vi "test_read-nmea-data2.vi"() -> ()   [LabVIEW 2019] (continued)
F9P\t\t\n15:10:07.17\tF9P\t\t\n15:10:07.19\tF9P\t\t\n15:10:07.21\tF9P\t\t\n15:10:07.23\tF9P\t\t\n15:10:07.25\tF9P\t$GNRMC,061009.00,A,3723.58159,N,12656.88383,E,1.806,,250720,,,A,V*1C\n\t\n15:10:07.27\tF9P\t$GNVTG,,T,,M,1.806,N,3.344,K,A*32\n\t\n15:10:07.29\tF9P\t$GNGGA,061009.00,3723.58159,N,12656.88383,E,1,12,0.64,44.5,M,18.5,M,,*7F\n\t\n15:10:07.31\tF9P\t$GNGSA,A,3,12,06,19,05,17,09,04,02,,,,,1.19,0.64,1.00,1*0A\n\t\n15:10:07.33\tF9P\t$GNGSA,A,3,85,71,84,,,,,,,,,,1.19,0.64,1.00,2*0F\n\t\n15:10:07.35\tF9P\t$GNGSA,A,3,36,19,11,04,09,12,,,,,,,1.19,0.64,1.00,3*0A\n\t\n15:10:07.37\tF9P\t$GNGSA,A,3,14,11,33,,,,,,,,,,1.19,0.64,1.00,4*0B\n\t\n15:10:07.39\tF9P\t$GPGSV,3,1,09,02,54,318,25,04,19,044,11,05,36,246,25,06,65,046,30,1*6E\n\t\n15:10:07.41\tF9P\t$GPGSV,3,2,09,09,45,075,26,12,24,278,18,17,34,153,25,19,53,156,23,1*6F\n\t\n15:10:07.43\tF9P\t$GPGSV,3,3,09,25,12,307,15,1*59\n\t\n15:10:07.45\tF9P\t$GPGSV,3,1,09,02,54,318,,04,19,044,,05,36,246,18,06,65,046,13,6*61\n\t\n15:10:07.47\tF9P\t$GPGSV,3,2,09,09,45,075,12,12,24,278,,17,34,153,,19,53,156,,6*60\n\t\n15:10:07.49\tF9P\t$GPGSV,3,3,09,25,12,307,,6*5A\n\t\n15:10:07.51\tF9P\t$GLGSV,2,1,08,69,12,031,,70,72,041,,71,51,205,19,72,03,209,,1*7A\n\t\n15:10:07.53\tF9P\t$GLGSV,2,2,08,77,01,327,,84,21,121,11,85,70,063,21,86,35,329,,1*76\n\t\n15:10:07.55\tF9P\t$GLGSV,2,1,08,69,12,031,,70,72,041,,71,51,205,28,72,03,209,,3*7A\n\t\n15:10:07.57\tF9P\t$GLGSV,2,2,08,77,01,327,,84,21,121,14,85,70,063,20,86,35,329,,3*70\n\t\n15:10:07.59\tF9P\t$GAGSV,2,1,08,02,09,298,10,04,66,119,24,09,31,193,15,11,71,357,22,7*79\n\t\n15:10:07.61\tF9P\t$GAGSV,2,2,08,12,40,102,18,19,27,045,22,25,09,249,,36,25,308,16,7*75\n\t\n15:10:07.63\tF9P\t$GAGSV,2,1,08,02,09,298,,04,66,119,20,09,31,193,,11,71,357,15,2*79\n\t\n15:10:07.65\tF9P\t$GAGSV,2,2,08,12,40,102,,19,27,045,,25,09,249,,36,25,308,,2*7E\n\t\n15:10:07.67\tF9P\t$GBGSV,1,1,03,11,50,131,19,14,87,138,20,33,60,219,25,1*42\n\t\n15:10:07.69\tF9P\t$GBGSV,1,1,03,11,50,131,16,14,87,138,22,33,60,219,,3*4A\n\t\n15:10:07.71\tF9P\t$GNGLL,3723.58159,N,12656.88383,E,061009.00,A,A*72\n\t\n15:10:07.73\tF9P\t\t\n15:10:07.75\tF9P\t\t\n15:10:07.77\tF9P\t\t\n15:10:07.79\tF9P\t\t\n15:10:07.81\tF9P\t\t\n15:10:07.83\tF9P\t\t\n15:10:07.85\tF9P\t\t\n15:10:07.87\tF9P\t\t\n15:10:07.89\tF9P\t\t\n15:10:07.91\tF9P\t\t\n15:10:07.93\tF9P\t\t\n15:10:07.95\tF9P\t\t\n15:10:07.97\tF9P\t\t\n15:10:07.99\tF9P\t\t\n15:10:08.01\tF9P\t\t\n15:10:08.03\tF9P\t\t\n15:10:08.05\tF9P\t\t\n15:10:08.07\tF9P\t\t\n15:10:08.09\tF9P\t\t\n15:10:08.11\tF9P\t\t\n15:10:08.13\tF9P\t\t\n15:10:08.15\tF9P\t\t\n15:10:08.17\tF9P\t\t\n15:10:08.19\tF9P\t\t\n15:10:08.21\tF9P\t\t\n15:10:08.23\tF9P\t\t\n15:10:08.25\tF9P\t$GNRMC,061010.00,A,3723.58119,N,12656.88346,E,1.587,,250720,,,A,V*1D\n\t\n15:10:08.27\tF9P\t$GNVTG,,T,,M,1.587,N,2.938,K,A*36\n\t\n15:10:08.29\tF9P\t$GNGGA,061010.00,3723.58119,N,12656.88346,E,1,12,0.64,46.1,M,18.5,M,,*7C\n\t\n15:10:08.31\tF9P\t$GNGSA,A,3,12,06,19,05,17,09,04,02,,,,,1.19,0.64,1.00,1*0A\n\t\n15:10:08.33\tF9P\t$GNGSA,A,3,85,71,84,,,,,,,,,,1.19,0.64,1.00,2*0F\n\t\n15:10:08.35\tF9P\t$GNGSA,A,3,36,19,11,04,09,12,,,,,,,1.19,0.64,1.00,3*0A\n\t\n15:10:08.37\tF9P\t$GNGSA,A,3,14,11,33,,,,,,,,,,1.19,0.64,1.00,4*0B\n\t\n15:10:08.39\tF9P\t$GPGSV,3,1,09,02,54,318,24,04,19,044,14,05,36,246,24,06,65,046,25,1*6F\n\t\n15:10:08.41\tF9P\t$GPGSV,3,2,09,09,45,075,33,12,24,278,19,17,34,153,23,19,53,156,23,1*6C\n\t\n15:10:08.43\tF9P\t$GPGSV,3,3,09,25,12,307,14,1*58\n\t\n15:10:08.45\tF9P\t$GPGSV,3,1,09,02,54,318,,04,19,044,,05,36,246,17,06,65,046,15,6*68\n\t\n15:10:08.47\tF9P\t$GPGSV,3,2,09,09,45,075,12,12,24,278,,17,34,153,,19,53,156,,6*60\n\t\n15:10:08.49\tF9P\t$GPGSV,3,3,09,25,12,307,,6*5A\n\t\n15:10:08.51\tF9P\t$GLGSV,2,1,08,69,12,031,,70,72,041,,71,51,205,18,72,03,209,,1*7B\n\t\n15:10:08.53\tF9P\t$GLGSV,2,2,08,77,01,327,,84,21,121,10,85,70,063,21,86,35,329,,1*77\n\t\n15:10:08.55\tF9P\t$GLGSV,2,1,08,69,12,031,,70,72,041,,71,51,205,27,72,03,209,,3*75\n\t\n15:10:08.57\tF9P\t$GLGSV,2,2,08,77,01,327,,84,21,121,13,85,70,063,20,86,35,329,,3*77\n\t\n15:10:08.59\tF9P\t$GAGSV,2,1,08,02,09,298,10,04,66,119,26,09,31,193,19,11,71,357,21,7*74\n\t\n15:10:08.61\tF9P\t$GAGSV,2,2,08,12,40,102,20,19,27,045,24,25,09,249,,36,25,308,18,7*76\n\t\n15:10:08.63\tF9P\t$GAGSV,2,1,08,02,09,298,,04,66,119,20,09,31,193,,11,71,357,16,2*7A\n\t\n15:10:08.65\tF9P\t$GAGSV,2,2,08,12,40,102,,19,27,045,,25,09,249,,36,25,308,,2*7E\n\t\n15:10:08.67\tF9P\t$GBGSV,1,1,03,11,50,131,19,14,87,138,21,33,60,219,26,1*40\n\t\n15:10:08.69\tF9P\t$GBGSV,1,1,03,11,50,131,18,14,87,138,22,33,60,219,,3*44\n\t\n15:10:08.71\tF9P\t$GNGLL,3723.58119,N,12656.88346,E,061010.00,A,A*77\n\t\n15:10:08.74\tF9P\t\t\n15:10:08.76\tF9P\t\t\n15:10:08.78\tF9P\t\t\n15:10:08.80\tF9P\t\t\n15:10:08.82\tF9P\t\t\n15:10:08.84\tF9P\t\t\n15:10:08.86\tF9P\t\t\n15:10:08.88\tF9P\t\t\n15:10:08.90\tF9P\t\t\n15:10:08.92\tF9P\t\t\n15:10:08.94\tF9P\t\t\n15:10:08.96\tF9P\t\t\n15:10:08.98\tF9P\t\t\n15:10:09.00\tF9P\t\t\n15:10:09.02\tF9P\t\t\n15:10:09.04\tF9P\t\t\n15:10:09.06\tF9P\t\t\n15:10:09.08\tF9P\t\t\n15:10:09.10\tF9P\t\t\n15:10:09.12\tF9P\t\t\n15:10:09.14\tF9P\t\t\n15:10:09.16\tF9P\t\t\n15:10:09.18\tF9P\t\t\n15:10:09.20\tF9P\t\t\n15:10:09.22\tF9P\t\t\n15:10:09.24\tF9P\t\t\n15:10:09.26\tF9P\t$GNRMC,061011.00,A,3723.58042,N,12656.88317,E,2.775,203.67,250720,,,A,V*05\n\t\n15:10:09.28\tF9P\t$GNVTG,203.67,T,,M,2.775,N,5.139,K,A*2A\n\t\n15:10:09.30\tF9P\t$GNGGA,061011.00,3723.58042,N,12656.88317,E,1,12,0.64,47.7,M,18.5,M,,*71\n\t\n15:10:09.32\tF9P\t$GNGSA,A,3,12,06,19,05,17,09,04,02,,,,,1.19,0.64,1.00,1*0A\n\t\n15:10:09.34\tF9P\t$GNGSA,A,3,85,71,84,,,,,,,,,,1.19,0.64,1.00,2*0F\n\t\n15:10:09.36\tF9P\t$GNGSA,A,3,36,19,11,04,09,12,,,,,,,1.19,0.64,1.00,3*0A\n\t\n15:10:09.38\tF9P\t$GNGSA,A,3,14,11,33,,,,,,,,,,1.19,0.64,1.00,4*0B\n\t\n15:10:09.40\tF9P\t$GPGSV,3,1,09,02,54,318,23,04,19,044,14,05,36,246,24,06,65,046,32,1*6E\n\t\n15:10:09.42\tF9P\t$GPGSV,3,2,09,09,45,075,33,12,24,278,18,17,34,153,23,19,53,156,24,1*6A\n\t\n15:10:09.44\tF9P\t$GPGSV,3,3,09,25,12,307,13,1*5F\n\t\n15:10:09.46\tF9P\t$GPGSV,3,1,09,02,54,318,,04,19,044,,05,36,246,18,06,65,046,15,6*67\n\t\n15:10:09.48\tF9P\t$GPGSV,3,2,09,09,45,075,,12,24,278,,17,34,153,,19,53,156,,6*63\n\t\n15:10:09.50\tF9P\t$GPGSV,3,3,09,25,12,307,,6*5A\n\t\n15:10:09.52\tF9P\t$GLGSV,2,1,08,69,12,031,,70,72,041,,71,51,205,18,72,03,209,,1*7B\n\t\n15:10:09.54\tF9P\t$GLGSV,2,2,08,77,01,327,,84,21,121,10,85,70,063,22,86,35,329,,1*74\n\t\n15:10:09.56\tF9P\t$GLGSV,2,1,08,69,12,031,,70,72,041,,71,51,205,26,72,03,209,,3*74\n\t\n15:10:09.58\tF9P\t$GLGSV,2,2,08,77,01,327,,84,21,121,18,85,70,063,20,86,35,329,,3*7C\n\t\n15:10:09.60\tF9P\t$GAGSV,2,1,08,02,09,298,10,04,66,119,26,09,31,193,19,11,71,357,21,7*74\n\t\n15:10:09.62\tF9P\t$GAGSV,2,2,08,12,40,102,21,19,27,045,24,25,09,249,,36,25,308,17,7*78\n\t\n15:10:09.64\tF9P\t$GAGSV,2,1,08,02,09,298,,04,66,119,20,09,31,193,,11,71,357,14,2*78\n\t\n15:10:09.66\tF9P\t$GAGSV,2,2,08,12,40,102,,19,27,045,,25,09,249,,36,25,308,,2*7E\n\t\n15:10:09.68\tF9P\t$GBGSV,1,1,03,11,50,131,18,14,87,138,20,33,60,219,26,1*40\n\t\n15:10:09.70\tF9P\t$GBGSV,1,1,03,11,50,131,18,14,87,138,21,33,60,219,,3*47\n\t\n15:10:09.72\tF9P\t$GNGLL,3723.58042,N,12656.88317,E,061011.00,A,A*7D\n\t\n15:10:09.74\tF9P\t\t\n15:10:09.76\tF9P\t\t\n15:10:09.78\tF9P\t\t\n15:10:09.80\tF9P\t\t\n15:10:09.82\tF9P\t\t\n15:10:09.84\tF9P\t\t\n15:10:09.86\tF9P\t\t\n15:10:09.88\tF9P\t\t\n15:10:09.90\tF9P\t\t\n15:10:09.92\tF9P\t\t\n15:10:09.94\tF9P\t\t\n15:10:09.96\tF9P\t\t\n15:10:09.98\tF9P\t\t\n15:10:10.00\tF9P\t\t\n15:10:10.02\tF9P\t\t\n15:10:10.04\tF9P\t\t\n15:10:10.06\tF9P\t\t\n15:10:10.08\tF9P\t\t\n15:10:10.10\tF9P\t\t\n15:10:10.12\tF9P\t\t\n15:10:10.14\tF9P\t\t\n15:10:10.16\tF9P\t\t\n15:10:10.18\tF9P\t\t\n15:10:10.20\tF9P\t\t\n15:10:10.22\tF9P\t\t\n15:10:10.24\tF9P\t\t\n15:10:10.26\tF9P\t$GNRMC,061012.00,A,3723.57986,N,12656.88305,E,1.614,,250720,,,A,V*10\n\t\n15:10:10.28\tF9P\t$GNVTG,,T,,M,1.614,N,2.989,K,A*35\n\t\n15:10:10.30\tF9P\t$GNGGA,061012.00,3723.57986,N,12656.88305,E,1,12,0.64,49.2,M,18.5,M,,*74\n\t\n15:10:10.32\tF9P\t$GNGSA,A,3,12,06,19,05,17,09,04,02,,,,,1.19,0.64,1.00,1*0A\n\t\n15:10:10.34\tF9P\t$GNGSA,A,3,85,71,84,,,,,,,,,,1.19,0.64,1.00,2*0F\n\t\n15:10:10.36\tF9P\t$GNGSA,A,3,36,19,11,04,09,12,,,,,,,1.19,0.64,1.00,3*0A\n\t\n15:10:10.38\tF9P\t$GNGSA,A,3,14,11,33,,,,,,,,,,1.19,0.64,1.00,4*0B\n\t\n15:10:10.40\tF9P\t$GPGSV,3,1,09,02,54,318,22,04,19,044,14,05,36,246,24,06,65,046,31,1*6C\n\t\n15:10:10.42\tF9P\t$GPGSV,3,2,09,09,45,075,20,12,24,278,19,17,34,153,22,19,53,156,22,1*6E\n\t\n15:10:10.44\tF9P\t$GPGSV,3,3,09,25,12,307,12,1*5E\n\t\n15:10:10.46\tF9P\t$GPGSV,3,1,09,02,54,318,,04,19,044,,05,36,246,18,06,65,046,16,6*64\n\t\n15:10:10.48\tF9P\t$GPGSV,3,2,09,09,45,075,,12,24,278,,17,34,153,,19,53,156,,6*63\n\t\n15:10:10.50\tF9P\t$GPGSV,3,3,09,25,12,307,,6*5A\n\t\n15:10:10.52\tF9P\t$GLGSV,2,1,08,69,12,031,,70,72,041,,71,51,205,17,72,03,209,,1*74\n\t\n15:10:10.54\tF9P\t$GLGSV,2,2,08,77,01,327,,84,21,121,10,85,70,063,23,86,35,329,,1*75\n\t\n15:10:10.56\tF9P\t$GLGSV,2,1,08,69,12,031,,70,72,041,,71,51,205,24,72,03,209,,3*76\n\t\n15:10:10.58\tF9P\t$GLGSV,2,2,08,77,01,327,,84,21,121,14,85,70,063,19,86,35,329,,3*7A\n\t\n15:10:10.60\tF9P\t$GAGSV,2,1,08,02,09,298,08,04,66,119,31,09,31,193,19,11,71,357,22,7*78\n\t\n15:10:10.62\tF9P\t$GAGSV,2,2,08,12,40,102,20,19,27,045,23,25,09,249,,36,25,308,18,7*71\n\t\n15:10:10.64\tF9P\t$GAGSV,2,1,08,02,09,298,,04,66,119,21,09,31,193,,11,71,357,15,2*78\n\t\n15:10:10.66\tF9P\t$GAGSV,2,2,08,12,40,102,,19,27,045,,25,09,249,,36,25,308,,2*7E\n\t\n15:10:10.68\tF9P\t$GBGSV,1,1,03,11,50,131,20,14,87,138,19,33,60,219,26,1*41\n\t\n15:10:10.70\tF9P\t$GBGSV,1,1,03,11,50,131,28,14,87,138,20,33,60,219,,3*45\n\t\n15:10:10.72\tF9P\t$GNGLL,3723.57986,N,12656.88305,E,061012.00,A,A*73\n\t\n15:10:10.74\tF9P\t\t\n15:10:10.76\tF9P\t\t\n15:10:10.78\tF9P\t\t\n15:10:10.80\tF9P\t\t\n15:10:10.82\tF9P\t\t\n15:10:10.84\tF9P\t\t\n15:10:10.86\tF9P\t\t\n15:10:10.88\tF9P\t\t\n15:10:10.90\tF9P\t\t\n15:10:10.92\tF9P\t\t\n15:10:10.94\tF9P\t\t\n15:10:10.96\tF9P\t\t\n15:10:10.98\tF9P\t\t\n15:10:11.00\tF9P\t\t\n15:10:11.02\tF9P\t\t\n15:10:11.04\tF9P\t\t\n15:10:11.06\tF9P\t\t\n15:10:11.08\tF9P\t\t\n15:10:11.10\tF9P\t\t\n15:10:11.12\tF9P\t\t\n15:10:11.14\tF9P\t\t\n15:10:11.16\tF9P\t\t\n15:10:11.18\tF9P\t\t\n15:10:11.20\tF9P\t\t\n15:10:11.22\tF9P\t\t\n15:10:11.24\tF9P\t$GNRMC,061013.00,A,3723.57921,N,12656.88315,E,2.275,191.13,250720,,,A,V*08\n\t\n15:10:11.26\tF9P\t$GNVTG,191.13,T,,M,2.275,N,4.213,K,A*2E\n\t\n15:10:11.28\tF9P\t$GNGGA,061013.00,3723.57921,N,12656.88315,E,1,12,0.64,50.6,M,18.5,M,,*75\n\t\n15:10:11.30\tF9P\t$GNGSA,A,3,12,06,19,05,17,09,04,02,,,,,1.19,0.64,1.00,1*0A\n\t\n15:10:11.32\tF9P\t$GNGSA,A,3,85,71,84,,,,,,,,,,1.19,0.64,1.00,2*0F\n\t\n15:10:11.34\tF9P\t$GNGSA,A,3,36,19,11,04,09,12,,,,,,,1.19,0.64,1.00,3*0A\n\t\n15:10:11.36\tF9P\t$GNGSA,A,3,14,11,33,,,,,,,,,,1.19,0.64,1.00,4*0B\n\t\n15:10:11.38\tF9P\t$GPGSV,3,1,09,02,54,318,29,04,19,044,13,05,36,246,25,06,65,046,26,1*67\n\t\n15:10:11.40\tF9P\t$GPGSV,3,2,09,09,45,075,29,12,24,278,20,17,34,153,21,19,53,156,22,1*6E\n\t\n15:10:11.42\tF9P\t$GPGSV,3,3,09,25,12,307,10,1*5C\n\t\n15:10:11.44\tF9P\t$GPGSV,3,1,09,02,54,318,,04,19,044,,05,36,246,17,06,65,046,15,6*68\n\t\n15:10:11.46\tF9P\t$GPGSV,3,2,09,09,45,075,,12,24,278,,17,34,153,,19,53,156,,6*63\n\t\n15:10:11.48\tF9P\t$GPGSV,3,3,09,25,12,307,,6*5A\n\t\n15:10:11.50\tF9P\t$GLGSV,2,1,08,69,12,031,,70,72,041,,71,51,205,16,72,03,209,,1*75\n\t\n15:10:11.52\tF9P\t$GLGSV,2,2,08,77,01,327,,84,21,121,09,85,70,063,22,86,35,329,,1*7C\n\t\n15:10:11.54\tF9P\t$GLGSV,2,1,08,69,12,031,,70,72,041,,71,51,205,24,72,03,209,,3*76\n\t\n15:10:11.56\tF9P\t$GLGSV,2,2,08,77,01,327,,84,21,121,14,85,70,063,21,86,35,329,,3*71\n\t\n15:10:11.58\tF9P\t$GAGSV,2,1,08,02,09,298,11,04,66,119,22,09,31,193,19,11,71,357,22,7*72\n\t\n15:10:11.60\tF9P\t$GAGSV,2,2,08,12,40,102,20,19,27,045,21,25,09,249,,36,25,308,16,7*7D\n\t\n15:10:11.62\tF9P\t$GAGSV,2,1,08,02,09,298,,04,66,119,20,09,31,193,,11,71,357,16,2*7A\n\t\n15:10:11.64\tF9P\t$GAGSV,2,2,08,12,40,102,,19,27,045,,25,09,249,,36,25,308,,2*7E\n\t\n15:10:11.66\tF9P\t$GBGSV,1,1,03,11,50,131,20,14,87,138,20,33,60,219,24,1*49\n\t\n15:10:11.68\tF9P\t$GBGSV,1,1,03,11,50,131,26,14,87,138,20,33,60,219,,3*4B\n\t\n15:10:11.70\tF9P\t$GNGLL,3723.57921,N,12656.88315,E,061013.00,A,A*7E\n\t\n15:10:11.72\tF9P\t\t\n15:10:11.74\tF9P\t\t\n15:10:11.76\tF9P\t\t\n15:10:11.78\tF9P\t\t\n15:10:11.80\tF9P\t\t\n15:10:11.82\tF9P\t\t\n15:10:11.84\tF9P\t\t\n15:10:11.86\tF9P\t\t\n15:10:11.88\tF9P\t\t\n15:10:11.90\tF9P\t\t\n15:10:11.92\tF9P\t\t\n15:10:11.94\tF9P\t\t\n15:10:11.96\tF9P\t\t\n15:10:11.98\tF9P\t\t\n15:10:12.00\tF9P\t\t\n15:10:12.02\tF9P\t\t\n15:10:12.04\tF9P\t\t\n15:10:12.06\tF9P\t\t\n15:10:12.08\tF9P\t\t\n15:10:12.10\tF9P\t\t\n15:10:12.12\tF9P\t\t\n15:10:12.14\tF9P\t\t\n15:10:12.16\tF9P\t\t\n15:10:12.18\tF9P\t\t\n15:10:12.20\tF9P\t\t\n15:10:12.22\tF9P\t\t\n15:10:12.24\tF9P\t$GNRMC,061014.00,A,3723.57868,N,12656.88291,E,1.974,,250720,,,A,V*12\n\t\n15:10:12.26\tF9P\t$GNVTG,,T,,M,1.974,N,3.656,K,A*30\n\t\n15:10:12.28\tF9P\t$GNGGA,061014.00,3723.57868,N,12656.88291,E,1,12,0.64,52.0,M,18.5,M,,*77\n\t\n15:10:12.31\tF9P\t$GNGSA,A,3,12,06,19,05,17,09,04,02,,,,,1.19,0.64,1.00,1*0A\n\t\n15:10:12.33\tF9P\t$GNGSA,A,3,85,71,84,,,,,,,,,,1.19,0.64,1.00,2*0F\n\t\n15:10:12.35\tF9P\t$GNGSA,A,3,36,19,11,04,09,12,,,,,,,1.19,0.64,1.00,3*0A\n\t\n15:10:12.37\tF9P\t$GNGSA,A,3,14,11,33,,,,,,,,,,1.19,0.64,1.00,4*0B\n\t\n15:10:12.39\tF9P\t$GPGSV,3,1,09,02,54,318,24,04,19,044,13,05,36,246,25,06,65,046,24,1*68\n\t\n15:10:12.41\tF9P\t$GPGSV,3,2,09,09,45,075,24,12,24,278,19,17,34,153,21,19,53,156,21,1*6A\n\t\n15:10:12.43\tF9P\t$GPGSV,3,3,09,25,12,307,,1*5D\n\t\n15:10:12.45\tF9P\t$GPGSV,3,1,09,02,54,318,,04,19,044,,05,36,246,17,06,65,046,17,6*6A\n\t\n15:10:12.47\tF9P\t$GPGSV,3,2,09,09,45,075,,12,24,278,,17,34,153,,19,53,156,,6*63\n\t\n15:10:12.49\tF9P\t$GPGSV,3,3,09,25,12,307,,6*5A\n\t\n15:10:12.51\tF9P\t$GLGSV,2,1,08,69,12,031,,70,72,041,,71,51,205,17,72,03,209,,1*74\n\t\n15:10:12.53\tF9P\t$GLGSV,2,2,08,77,01,326,,84,21,121,09,85,70,063,21,86,35,329,,1*7E\n\t\n15:10:12.55\tF9P\t$GLGSV,2,1,08,69,12,031,,70,72,041,,71,51,205,22,72,03,209,,3*70\n\t\n15:10:12.57\tF9P\t$GLGSV,2,2,08,77,01,326,,84,21,121,13,85,70,063,21,86,35,329,,3*77\n\t\n15:10:12.59\tF9P\t$GAGSV,2,1,08,02,09,298,09,04,66,119,28,09,31,193,19,11,71,357,22,7*71\n\t\n15:10:12.61\tF9P\t$GAGSV,2,2,08,12,40,102,19,19,27,045,19,25,09,249,,36,25,308,14,7*7E\n\t\n15:10:12.63\tF9P\t$GAGSV,2,1,08,02,09,298,,04,66,119,21,09,31,193,,11,71,357,15,2*78\n\t\n15:10:12.65\tF9P\t$GAGSV,2,2,08,12,40,102,,19,27,045,,25,09,249,,36,25,308,,2*7E\n\t\n15:10:12.67\tF9P\t$GBGSV,1,1,03,11,50,131,22,14,87,138,21,33,60,219,23,1*4D\n\t\n15:10:12.69\tF9P\t$GBGSV,1,1,03,11,50,131,,14,87,138,22,33,60,219,,3*4D\n\t\n15:10:12.71\tF9P\t$GNGLL,3723.57868,N,12656.88291,E,061014.00,A,A*78\n\t\n15:10:12.73\tF9P\t\t\n15:10:12.75\tF9P\t\t\n15:10:12.77\tF9P\t\t\n15:10:12.79\tF9P\t\t\n15:10:12.81\tF9P\t\t\n15:10:12.83\tF9P\t\t\n15:10:12.85\tF9P\t\t\n15:10:12.87\tF9P\t\t\n15:10:12.89\tF9P\t\t\n15:10:12.91\tF9P\t\t\n15:10:12.93\tF9P\t\t\n15:10:12.95\tF9P\t\t\n15:10:12.97\tF9P\t\t\n15:10:12.99\tF9P\t\t\n15:10:13.01\tF9P\t\t\n15:10:13.03\tF9P\t\t\n15:10:13.05\tF9P\t\t\n15:10:13.07\tF9P\t\t\n15:10:13.09\tF9P\t\t\n15:10:13.11\tF9P\t\t\n15:10:13.13\tF9P\t\t\n15:10:13.15\tF9P\t\t\n15:10:13.17\tF9P\t\t\n15:10:13.19\tF9P\t\t\n15:10:13.21\tF9P\t\t\n15:10:13.23\tF9P\t\t\n15:10:13.25\tF9P\t$GNRMC,061015.00,A,3723.57806,N,12656.88324,E,2.260,168.28,250720,,,A,V*02\n\t\n15:10:13.27\tF9P\t$GNVTG,168.28,T,,M,2.260,N,4.185,K,A*28\n\t\n15:10:13.29\tF9P\t$GNGGA,061015.00,3723.57806,N,12656.88324,E,1,12,0.64,52.7,M,18.5,M,,*76\n\t\n15:10:13.31\tF9P\t$GNGSA,A,3,12,06,19,05,17,09,04,02,,,,,1.19,0.64,1.00,1*0A\n\t\n15:10:13.33\tF9P\t$GNGSA,A,3,85,71,84,,,,,,,,,,1.19,0.64,1.00,2*0F\n\t\n15:10:13.35\tF9P\t$GNGSA,A,3,36,19,11,04,09,12,,,,,,,1.19,0.64,1.00,3*0A\n\t\n15:10:13.37\tF9P\t$GNGSA,A,3,14,11,33,,,,,,,,,,1.19,0.64,1.00,4*0B\n\t\n15:10:13.39\tF9P\t$GPGSV,3,1,09,02,54,318,25,04,19,044,12,05,36,246,25,06,65,046,25,1*69\n\t\n15:10:13.41\tF9P\t$GPGSV,3,2,09,09,45,075,27,12,24,278,19,17,34,153,23,19,53,156,22,1*68\n\t\n15:10:13.43\tF9P\t$GPGSV,3,3,09,25,12,307,,1*5D\n\t\n15:10:13.45\tF9P\t$GPGSV,3,1,09,02,54,318,,04,19,044,,05,36,246,16,06,65,046,17,6*6B\n\t\n15:10:13.47\tF9P\t$GPGSV,3,2,09,09,45,075,,12,24,278,,17,34,153,,19,53,156,,6*63\n\t\n15:10:13.49\tF9P\t$GPGSV,3,3,09,25,12,307,,6*5A\n\t\n15:10:13.51\tF9P\t$GLGSV,2,1,08,69,12,031,,70,72,041,,71,51,205,18,72,03,209,,1*7B\n\t\n15:10:13.53\tF9P\t$GLGSV,2,2,08,77,01,326,,84,21,121,12,85,70,063,21,86,35,329,,1*74\n\t\n15:10:13.55\tF9P\t$GLGSV,2,1,08,69,12,031,,70,72,041,,71,51,205,22,72,03,209,,3*70\n\t\n15:10:13.57\tF9P\t$GLGSV,2,2,08,77,01,326,,84,21,121,12,85,70,063,20,86,35,329,,3*77\n\t\n15:10:13.59\tF9P\t$GAGSV,2,1,08,02,09,298,08,04,66,119,22,09,31,193,17,11,71,357,22,7*74\n\t\n15:10:13.61\tF9P\t$GAGSV,2,2,08,12,40,102,16,19,27,045,16,25,09,249,,36,25,308,14,7*7E\n\t\n15:10:13.63\tF9P\t$GAGSV,2,1,08,02,09,298,,04,66,119,23,09,31,193,,11,71,357,16,2*79\n\t\n15:10:13.65\tF9P\t$GAGSV,2,2,08,12,40,102,,19,27,045,,25,09,249,,36,25,308,,2*7E\n\t\n15:10:13.67\tF9P\t$GBGSV,1,1,03,11,50,131,22,14,87,138,20,33,60,219,21,1*4E\n\t\n15:10:13.69\tF9P\t$GBGSV,1,1,03,11,50,131,32,14,87,138,20,33,60,219,,3*4E\n\t\n15:10:13.71\tF9P\t$GNGLL,3723.57806,N,12656.88324,E,061015.00,A,A*7E\n\t\n15:10:13.73\tF9P\t\t\n15:10:13.75\tF9P\t\t\n15:10:13.77\tF9P\t\t\n15:10:13.79\tF9P\t\t\n15:10:13.81\tF9P\t\t\n15:10:13.83\tF9P\t\t\n15:10:13.85\tF9P\t\t\n15:10:13.87\tF9P\t\t\n15:10:13.89\tF9P\t\t\n15:10:13.91\tF9P\t\t\n15:10:13.93\tF9P\t\t\n15:10:13.95\tF9P\t\t\n15:10:13.97\tF9P\t\t\n15:10:13.99\tF9P\t\t\n15:10:14.01\tF9P\t\t\n15:10:14.03\tF9P\t\t\n15:10:14.05\tF9P\t\t\n15:10:14.07\tF9P\t\t\n15:10:14.09\tF9P\t\t\n15:10:14.11\tF9P\t\t\n15:10:14.13\tF9P\t\t\n15:10:14.15\tF9P\t\t\n15:10:14.17\tF9P\t\t\n15:10:14.19\tF9P\t\t\n15:10:14.21\tF9P\t\t\n15:10:14.23\tF9P\t\t\n15:10:14.25\tF9P\t$GNRMC,061016.00,A,3723.57737,N,12656.88342,E,2.502,169.99,250720,,,A,V*04\n\t\n15:10:14.27\tF9P\t$GNVTG,169.99,T,,M,2.502,N,4.634,K,A*2D\n\t\n15:10:14.29\tF9P\t$GNGGA,061016.00,3723.57737,N,12656.88342,E,1,12,0.64,53.9,M,18.5,M,,*77\n\t\n15:10:14.31\tF9P\t$GNGSA,A,3,12,06,19,05,17,09,04,02,,,,,1.19,0.64,1.00,1*0A\n\t\n15:10:14.33\tF9P\t$GNGSA,A,3,85,71,84,,,,,,,,,,1.19,0.64,1.00,2*0F\n\t\n15:10:14.35\tF9P\t$GNGSA,A,3,36,19,11,04,09,12,,,,,,,1.19,0.64,1.00,3*0A\n\t\n15:10:14.37\tF9P\t$GNGSA,A,3,14,11,33,,,,,,,,,,1.19,0.64,1.00,4*0B\n\t\n15:10:14.39\tF9P\t$GPGSV,3,1,09,02,54,318,24,04,19,044,10,05,36,246,25,06,65,046,25,1*6A\n\t\n15:10:14.41\tF9P\t$GPGSV,3,2,09,09,45,075,28,12,24,278,18,17,34,153,22,19,53,156,22,1*67\n\t\n15:10:14.43\tF9P\t$GPGSV,3,3,09,25,12,307,,1*5D\n\t\n15:10:14.45\tF9P\t$GPGSV,3,1,09,02,54,318,,04,19,044,,05,36,246,16,06,65,046,16,6*6A\n\t\n15:10:14.47\tF9P\t$GPGSV,3,2,09,09,45,075,,12,24,278,,17,34,153,,19,53,156,,6*63\n\t\n15:10:14.49\tF9P\t$GPGSV,3,3,09,25,12,307,,6*5A\n\t\n15:10:14.51\tF9P\t$GLGSV,2,1,08,69,12,031,,70,72,041,,71,51,205,18,72,03,209,,1*7B\n\t\n15:10:14.53\tF9P\t$GLGSV,2,2,08,77,01,326,,84,21,121,11,85,70,063,22,86,35,329,,1*74\n\t\n15:10:14.55\tF9P\t$GLGSV,2,1,08,69,12,031,,70,72,041,,71,51,205,22,72,03,209,,3*70\n\t\n15:10:14.57\tF9P\t$GLGSV,2,2,08,77,01,326,,84,21,121,11,85,70,063,19,86,35,329,,3*7E\n\t\n15:10:14.59\tF9P\t$GAGSV,2,1,08,02,09,298,11,04,66,119,22,09,31,193,17,11,71,357,22,7*7C\n\t\n15:10:14.61\tF9P\t$GAGSV,2,2,08,12,40,102,15,19,27,045,14,25,09,249,,36,25,308,14,7*7F\n\t\n15:10:14.63\tF9P\t$GAGSV,2,1,08,02,09,298,,04,66,119,21,09,31,193,,11,71,357,18,2*75\n\t\n15:10:14.65\tF9P\t$GAGSV,2,2,08,12,40,102,,19,27,045,,25,09,249,,36,25,308,,2*7E\n\t\n15:10:14.67\tF9P\t$GBGSV,1,1,03,11,50,131,23,14,87,138,21,33,60,219,22,1*4D\n\t\n15:10:14.69\tF9P\t$GBGSV,1,1,03,11,50,131,24,14,87,138,20,33,60,219,,3*49\n\t\n15:10:14.71\tF9P\t$GNGLL,3723.57737,N,12656.88342,E,061016.00,A,A*70\n\t\n15:10:14.73\tF9P\t\t\n15:10:14.75\tF9P\t\t\n15:10:14.77\tF9P\t\t\n15:10:14.79\tF9P\t\t\n
